vi "dds9954_interface_v2013.vi"(1 "DDS9954 Interface":T1, 2 "Previous Ascii Array In":string[](array[string])) -> (16 "Last Ascii array Out":string[](array[string]), 17 "Characters to FPGA":string="L;004\r\nL102200242\r\nL2000034\r\nL01\r\nL411<71<720::::::;0::::::;071<71<7\r\nL615555555155555550>38>38>0>38>38>\r\nL31000100010001000\r\nL50000000000000000\r\nL70200000001010000000102000000010200000001\r\nL80200000001010000000102000000010200000001\r\nL:0;>;<2000;>;<2000;>;<2000;>;<200\r\nL91010\r\n")   [LabVIEW 2013, in "DDS9954_v2013.lvlib"]
uses:
  DDS9954_v2013.lvlib
  dataToAscii_32bit.vi
panel:
  out "length":i32[](array[numeric])
  # "Data writing time:\n--Freq0 changed:  ~1.7 us\n--Amp changed:  ~1 us\n--Phase changed:  ~1 us\n--Sweep time changed:  ~3.4 us\n--ALL parameters changed:  ~9 us"
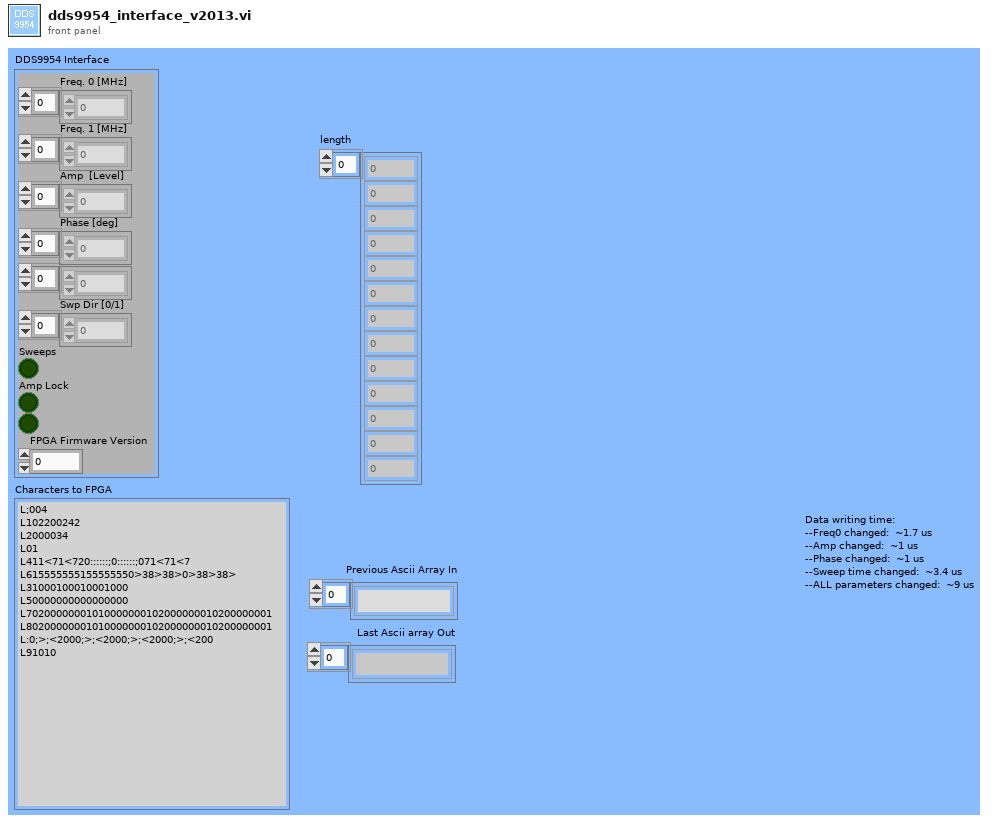
[diagram p1: front panel]
types:
  T1 = cluster{"Freq. 0 [MHz]":dbl[], "Freq. 1 [MHz]":dbl[], "Amp  [Level]":dbl[], "Phase [deg]":dbl[], dbl[], "Swp Dir [0/1]":u16[], "Sweeps":bool, "Amp Lock":bool, bool, "FPGA Firmware Version":dbl}
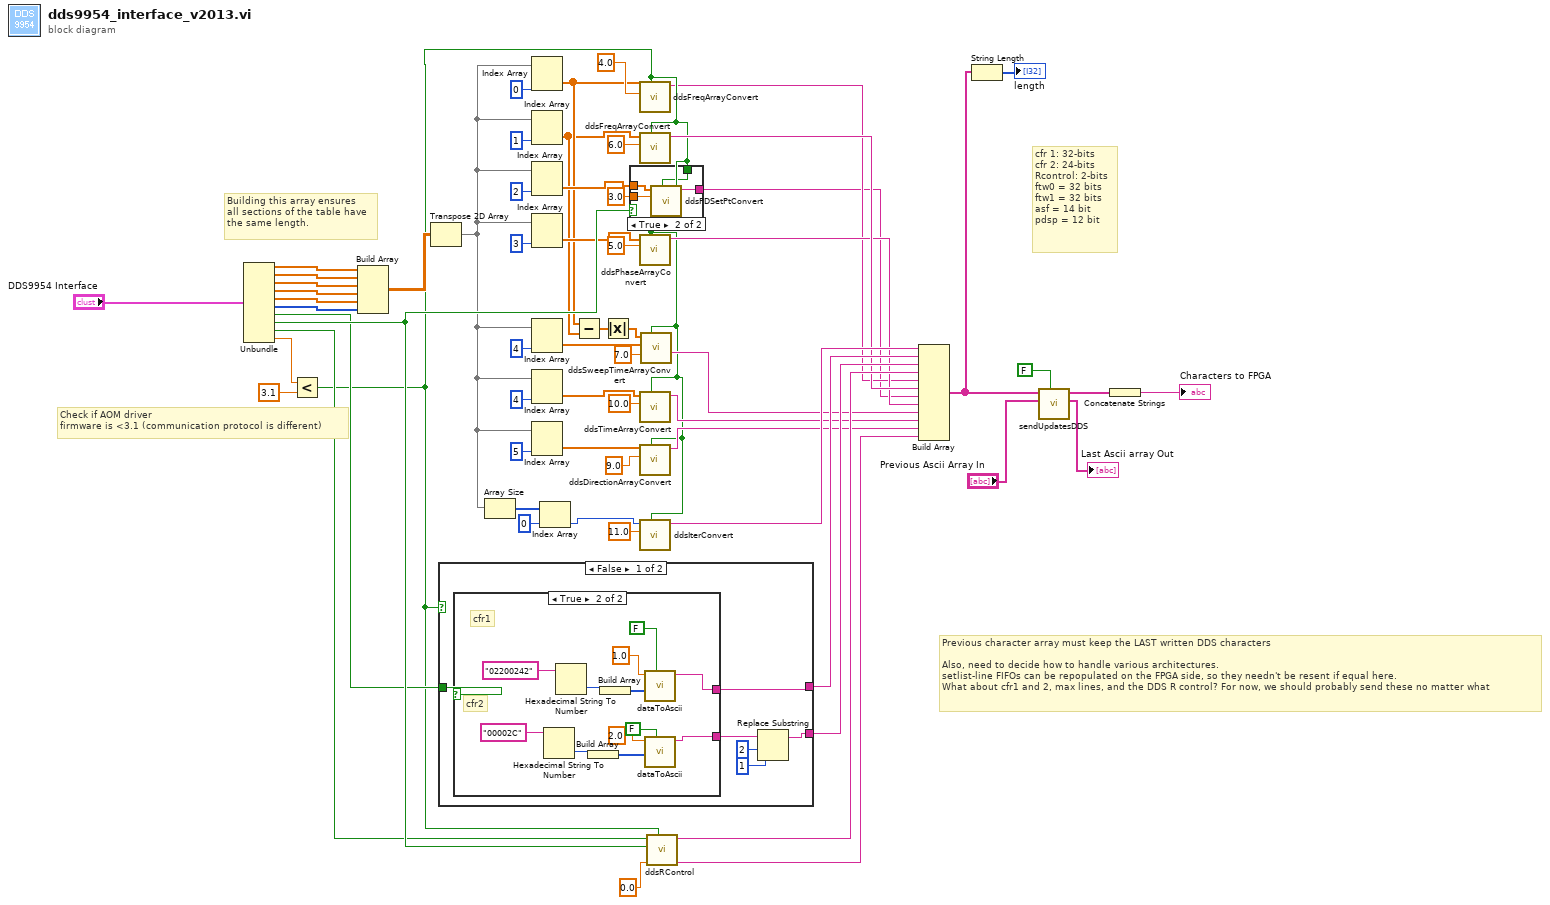
[diagram p0: block diagram]
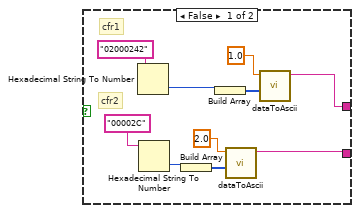
[diagram p2: hidden frame]
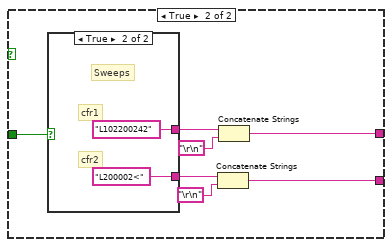
[diagram p3: hidden frame]
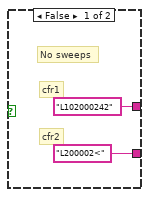
[diagram p4: hidden frame]
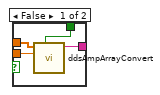
[diagram p5: hidden frame]
diagram:
  # "Check if AOM driver\nfirmware is <3.1 (communication protocol is different)"
  # "cfr 1: 32-bits\ncfr 2: 24-bits\nRcontrol: 2-bits\nftw0 = 32 bits\nftw1 = 32 bits\nasf = 14 bit\npdsp = 12 bit"
  # "Previous character array must keep the LAST written DDS characters\n\nAlso, need to decide how to handle various architectures.\nsetlist-line FIFOs can be repopulated on the FPGA side, so they needn't be resent if equal here.\nWhat about cfr1 and 2, max lines, and the DDS R control? For now, we should probably send these no matter what"
  # "Building this array ensures\nall sections of the table have\nthe same length."
  n1 = Unbundle("DDS9954 Interface") -> ("Freq. 0 [MHz]"=w54:dbl[], "Freq. 1 [MHz]"=w53:dbl[], "Amp  [Level]"=w52:dbl[], "Phase [deg]"=w51:dbl[], w50:dbl[], "Swp Dir [0/1]"=w49:u16[], "Sweeps"=w57:bool, "Amp Lock"=w62:bool, w58:bool, "FPGA Firmware Version"=w8:dbl)
  n2 = Less?(x=w8, y=3.1) -> (x < y?=w6:bool)
  n3 = Build Array(w54, w53, w52, w51, w50, w49) -> (w59:dbl[][])
  n4 = Transpose 2D Array(2D array=w59) -> (transposed array=w56:dbl[][])
  n5 = case shown="False" w6 {
    tunnel: w57 -> [w68 w97]
    tunnel: [w67 w92] -> w22
    tunnel: [w64 w91] -> w21
    frame False {
      n6 = case shown="True" w68 {
        tunnel: [w74 w86] -> w67
        tunnel: [w69 w81] -> w65
        frame False {
          # "cfr2"
          # "cfr1"
          n7 = Hexadecimal String To Number(string="02000242") -> (number=w77:u32)  [unwired: 2 in, 1 out]
          n8 = Hexadecimal String To Number(string="00002C") -> (number=w71:u32)  [unwired: 2 in, 1 out]
          n9 = Build Array(w71) -> (w73:u32[])
          n10 = Build Array(w77) -> (w78:u32[])
          n11 = call-poly "dataToAscii.vi"("Input Data"=w73, "Register"=2.0) -> ("Characters to FPGA"=w69:string)  [unwired: 9 in]
          n12 = call-poly "dataToAscii.vi"("Input Data"=w78, "Register"=1.0) -> ("Characters to FPGA"=w74:string)  [unwired: 9 in]
        }
        frame True {
          # "cfr2"
          # "cfr1"
          n13 = Hexadecimal String To Number(string="00002C") -> (number=w84:u32)  [unwired: 2 in, 1 out]
          n14 = Hexadecimal String To Number(string="02200242") -> (number=w89:u32)  [unwired: 2 in, 1 out]
          n15 = Build Array(w84) -> (w82:u32[])
          n16 = Build Array(w89) -> (w90:u32[])
          n17 = call-poly "dataToAscii.vi"("Pre 3.0 AOM driver version?"=FALSE, "Input Data"=w90, "Register"=1.0) -> ("Characters to FPGA"=w86:string)  [unwired: 8 in]
          n18 = call-poly "dataToAscii.vi"("Pre 3.0 AOM driver version?"=FALSE, "Input Data"=w82, "Register"=2.0) -> ("Characters to FPGA"=w81:string)  [unwired: 8 in]
        }
      }
      n19 = Replace Substring(2:1 ("length (len. of substring)"), 3:2 ("offset (0)"), 5:w65) -> (1:w64:string)  [unwired: 1 in, 1 out]
    }
    frame True {
      n20 = case shown="True" w97 {
        tunnel: ["L102000242" "L102200242"] -> w94
        tunnel: ["L200002<" "L200002<"] -> w93
        frame False {
          # "No sweeps"
          # "cfr2"
          # "cfr1"
        }
        frame True {
          # "Sweeps"
          # "cfr2"
          # "cfr1"
        }
      }
      n21 = Concatenate Strings(w93, "\r\n") -> (w91:string)
      n22 = Concatenate Strings(w94, "\r\n") -> (w92:string)
    }
  }
  n23 = Array Size(array=w56) -> (size(s)=w30:i32[])
  n24 = Index Array(array=w56, index (col)=0 ("disabled index (col)")) -> (element=w34:dbl[])  [unwired: 1 in]
  n25 = Index Array(array=w56, index (col)=1 ("disabled index (col)")) -> (element=w33:dbl[])  [unwired: 1 in]
  n26 = Index Array(array=w56, index (col)=2 ("disabled index (col)")) -> (element=w61:dbl[])  [unwired: 1 in]
  n27 = Index Array(array=w56, index (col)=3 ("disabled index (col)")) -> (element=w40:dbl[])  [unwired: 1 in]
  n28 = Index Array(array=w56, index (col)=4 ("disabled index (col)")) -> (element=w32:dbl[])  [unwired: 1 in]
  n29 = Index Array(array=w56, index (col)=4 ("disabled index (col)")) -> (element=w35:dbl[])  [unwired: 1 in]
  n30 = Index Array(array=w56, index (col)=5 ("disabled index (col)")) -> (element=w37:dbl[])  [unwired: 1 in]
  n31 = Index Array(array=w30, index=0) -> (element=w28:i32)
  n32 = Subtract(x=w34, y=w33) -> (x-y=w25:dbl[])
  n33 = Absolute Value(x=w25) -> (abs(x)=w24:dbl[])
  n34 = case shown="True" w62 {
    tunnel: 3.0 ("Register") -> [w104 w108]
    tunnel: w61 -> [w105 w109]
    tunnel: [w103 w107] -> w4
    tunnel: w6 -> [w102 w106]
    frame False {
      n35 = call "ddsAmpArrayConvert.vi"("Pre 3.0 AOM driver version?"=w102, "Register"=w104, "Amplitude Array (0-1)"=w105) -> ("Characters for FPGA"=w103:string)  [unwired: 8 in]
    }
    frame True {
      n36 = call "ddsPDSetPtConvert.vi"("Pre 3.0 AOM driver version?"=w106, "Register"=w108, "PD Set-Point (V)"=w109) -> ("Characters for FPGA"=w107:string)  [unwired: 8 in]
    }
  }
  n37 = call "ddsFreqArrayConvert.vi"("Pre 3.0 AOM driver version?"=w6, "Register"=4.0, "Frequency Array (MHz)"=w34) -> ("Characters for FPGA"=w5:string)  [unwired: 8 in]
  n38 = call "ddsFreqArrayConvert.vi"("Pre 3.0 AOM driver version?"=w6, "Register"=6.0, "Frequency Array (MHz)"=w33) -> ("Characters for FPGA"=w19:string)  [unwired: 8 in]
  n39 = call "ddsPhaseArrayConvert.vi"("Pre 3.0 AOM driver version?"=w6, "Register"=5.0, "Phase Array (degrees)"=w40) -> ("Characters for FPGA"=w18:string)  [unwired: 8 in]
  n40 = call "ddsTimeArrayConvert.vi"("Pre 3.0 AOM driver version?"=w6, "Register"=10.0, "Time Array (ms)"=w35) -> ("Characters for FPGA"=w16:string)  [unwired: 8 in]
  n41 = call "ddsDirectionArrayConvert.vi"("Pre 3.0 AOM driver version?"=w6, "Register"=9.0, "Direction (0 = down; 1 = up)"=w37) -> ("Characters for FPGA"=w15:string)  [unwired: 8 in]
  n42 = call "ddsIterConvert.vi"("Pre 3.0 AOM driver version?"=w6, "Register"=11.0, "Max Iterations"=w28) -> ("Characters for FPGA"=w23:string)  [unwired: 8 in]
  n43 = call "ddsSweepTimeArrayConvert.vi"("Pre 3.0 AOM driver"=w6, "Register"=7.0 ("N Register"), "Sweep Time Array (ms)"=w32, "Frequency Difference Array (MHz)"=w24) -> ("Characters for FPGA"=w17:string)  [unwired: 7 in]
  n44 = call "ddsRControl.vi"("Pre 3.0 AOM driver version?"=w6, "Register"=0.0, "Lock Amp"=w62, "Table/Sequence"=w58) -> ("Software Trigger"=w14:string, "Characters for FPGA"=w20:string)  [unwired: 6 in]
  n45 = Build Array(w23, w22, w21, w20, w5, w19, w4, w18, w17, w16, w15, w14) -> (w3:string[])
  n46 = String Length(string=w3) -> (length=→"length":i32[])
  n47 = call "sendUpdatesDDS.vi"("DDS: ProgramChanges"=FALSE, "Previous Ascii Array In"="Previous Ascii Array In", "Current Ascii Array In"=w3) -> ("Last written Ascii array Out"=→"Last Ascii array Out":string[], "Current Ascii Array Out"=w11:string[])  [unwired: 7 in]
  n48 = Concatenate Strings(w11) -> (→"Characters to FPGA":string)
